vi "Set_DL_Detector.vi"(8 "error in (no error)":errorcluster, 11 "Control-Server in":refnum<class "Control-Server.lvclass">) -> (0 "error out":errorcluster, 3 "Control-Server out":refnum<class "Control-Server.lvclass">)   [LabVIEW 2015, in "Control-Server.lvclass"]
uses:
  Control-Server.lvclass
  Config/config_names_def.ctl
  Delay Line/DelayLine.lvclass
  Delay Line/DelayLineLS4/DelayLineLS4.lvclass
  Delay Line/DelayLineOwis/DelayLineOwis.lvclass
  Detector/Detector.lvclass
  Detector/VIS-IR/VIS-NIR.lvclass
  Detector/UV-VIS/UV-VIS.lvclass
  dependecies/ControlsVIs/Clusters-def/UserEvent.ctl
  dependecies/ControlsVIs/Clusters-def/Message types.ctl
  Message/Message.lvclass
  Message/Message.lvclass/Message.ctl
  GeneralFunctionality/GeneralFunctionality.lvclass/GeneralFunctionality.ctl
  dependecies/ControlsVIs/Clusters-def/list-of-keys-DAQmx-tasks.ctl
  Control-Server.lvclass/Control-Server.ctl
  Detector/Detector.lvclass/Detector.ctl
  Config/Config.lvclass
  GeneralFunctionality/GeneralFunctionality.lvclass
  DAQmxTasks/DAQmxTaskContainer/DAQmxTaskContainer.lvclass
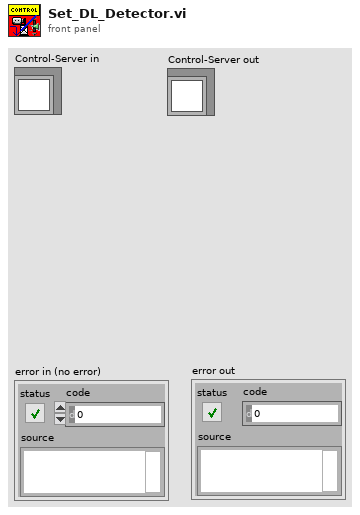
[diagram p1: front panel]
types:
  T1 = typedef "Config.lvclass/config_names_def.ctl" = string
  T2 = typedef "Message types.ctl" = string
  T3 = typedef "UserEvent.ctl" = cluster{"command":string, "data":variant}
  T4 = typedef "DAQmxTaskContainer.lvclass/list-of-keys-DAQmx-tasks.ctl" = string
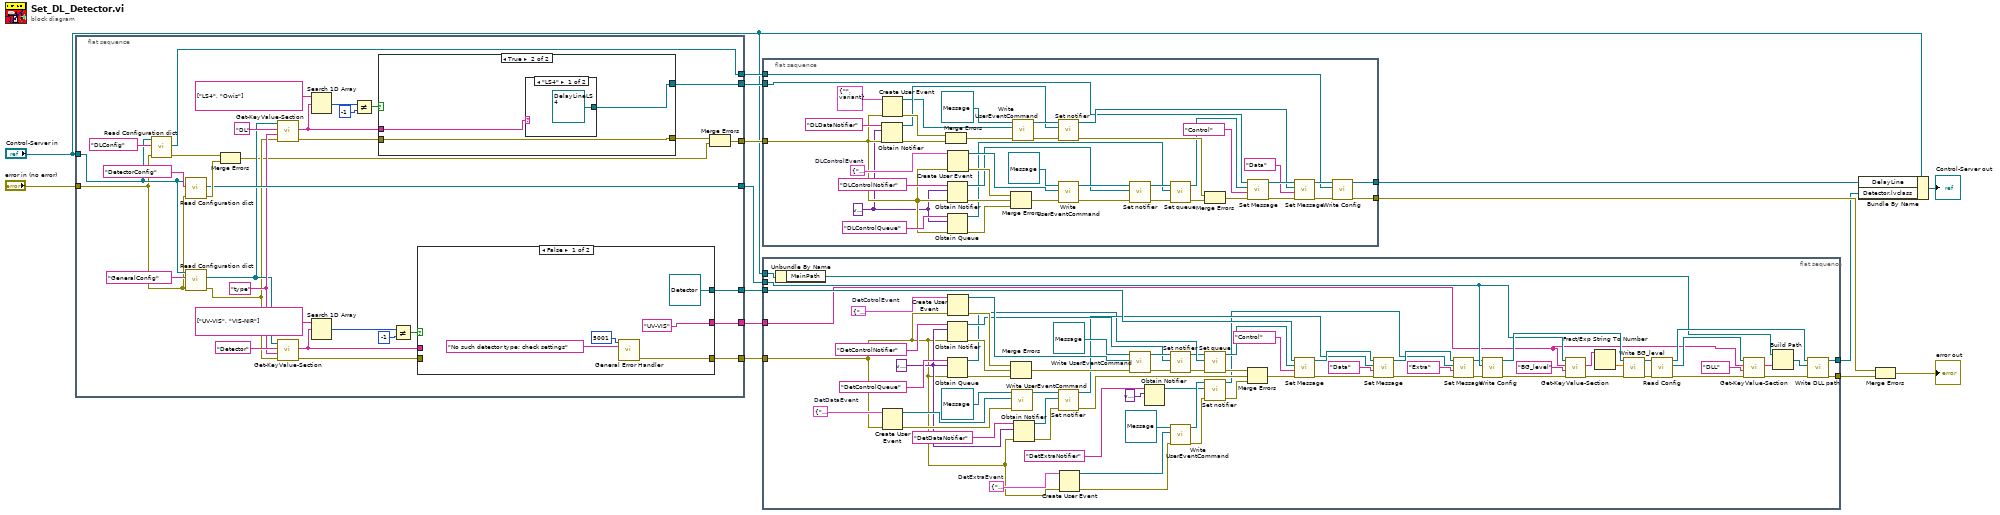
[diagram p0: block diagram]
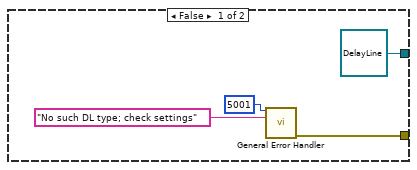
[diagram p2: hidden frame]
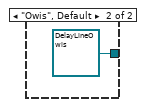
[diagram p3: hidden frame]
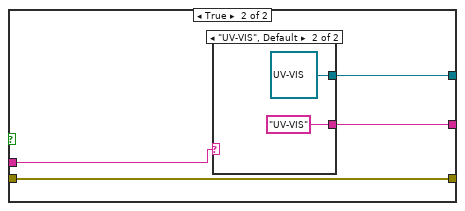
[diagram p4: hidden frame]
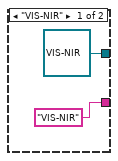
[diagram p5: hidden frame]
diagram:
  n1 = flat-sequence {
    tunnel: "Control-Server in" -> [w32]
    tunnel: "error in (no error)" -> [w31]
    tunnel: [w36] -> w9
    tunnel: [w18] -> w10
    tunnel: [w35] -> w11
    tunnel: [w34] -> w12
    tunnel: [w33] -> w13
    tunnel: [w27] -> w15
    tunnel: [w16] -> w1
    frame #0 {
      w25 = "type" ("Key")
      n2 = call "Read Configuration dict.vi"("error in (no error)"=w31, "Config Name"=T1 "DLConfig", "Control in"=w32) -> ("error out"=w38:errorcluster, "Config"=w36:refnum<class "Config.lvclass">)  [unwired: 6 in, 1 out]
      n3 = call "Read Configuration dict.vi"("error in (no error)"=w31, "Config Name"=T1 "DetectorConfig", "Control in"=w32) -> ("error out"=w37:errorcluster, "Config"=w35:refnum<class "Config.lvclass">)  [unwired: 6 in, 1 out]
      n4 = call "Read Configuration dict.vi"("error in (no error)"=w31, "Config Name"=T1 "GeneralConfig", "Control in"=w32) -> ("error out"=w22:errorcluster, "Config"=w23:refnum<class "Config.lvclass">)  [unwired: 6 in, 1 out]
      n5 = Merge Errors(w38, w37) -> (w20:errorcluster)
      n6 = call-dynamic "Get-KeyValue-Section.vi"("error in (no error)"=w22, "Key"=w25, "Section"="DL", "Config in"=w23) -> ("error out"=w21:errorcluster, "Value"=w17:string)  [unwired: 5 in, 1 out]
      n7 = call-dynamic "Get-KeyValue-Section.vi"("error in (no error)"=w22, "Key"=w25, "Section"="Detector", "Config in"=w23) -> ("error out"=w41:errorcluster, "Value"=w42:string)  [unwired: 5 in, 1 out]
      n8 = Search 1D Array(1D array=string[] ["LS4", "Owis"], element=w17) -> (index of element=w29:i32)  [unwired: 1 in]
      n9 = Search 1D Array(1D array=string[] ["UV-VIS", "VIS-NIR"], element=w42) -> (index of element=w45:i32)  [unwired: 1 in]
      n10 = Not Equal?(x=w29, y=-1) -> (x != y?=w28:bool)
      n11 = case shown="True" w28 {
        tunnel: [w50 w54] -> w19
        tunnel: [refnum<class "DelayLine.lvclass"> refnum ("DelayLine.lvclass") w55] -> w27
        tunnel: w21 -> [_ w54]
        tunnel: w17 -> [_ w53]
        frame False {
          n12 = call <vilib>:"General Error Handler.vi"("[error code] (0)"=5001 ("code"), "[error source] (\" \")"="No such DL type; check settings" ("String to Prepend to source (\"\")")) -> ("error out"=w50:errorcluster)  [unwired: 9 in, 4 out]
        }
        frame True {
          n13 = case shown="\"LS4\"" w53 {
            tunnel: [refnum<class "DelayLineLS4.lvclass"> refnum ("DelayLineLS4.lvclass") refnum<class "DelayLineOwis.lvclass"> refnum ("DelayLineOwis.lvclass")] -> w55
            frame "LS4" {
            }
            frame "Owis", Default {
            }
          }
        }
      }
      n14 = Not Equal?(x=w45, y=-1) -> (x != y?=w43:bool)
      n15 = case shown="False" w43 {
        tunnel: w42 -> [_ w66]
        tunnel: [refnum<class "Detector.lvclass"> refnum ("Detector.lvclass") w64] -> w33
        tunnel: w41 -> [_ w65]
        tunnel: [w59 w65] -> w34
        tunnel: ["UV-VIS" ("Section") w63] -> w16
        frame False {
          n16 = call <vilib>:"General Error Handler.vi"("[error code] (0)"=5001 ("code"), "[error source] (\" \")"="No such detector type; check settings" ("String to Prepend to source (\"\")")) -> ("error out"=w59:errorcluster)  [unwired: 9 in, 4 out]
        }
        frame True {
          n17 = case shown="\"UV-VIS\", Default" w66 {
            tunnel: [refnum<class "VIS-NIR.lvclass"> refnum ("VIS-IR.lvclass") refnum<class "UV-VIS.lvclass"> refnum ("UV-VIS.lvclass")] -> w64
            tunnel: ["VIS-NIR" ("Section") "UV-VIS" ("Section")] -> w63
            frame "VIS-NIR" {
            }
            frame "UV-VIS", Default {
            }
          }
        }
      }
      n18 = Merge Errors(w19, w20) -> (w18:errorcluster)
    }
  }
  n19 = flat-sequence {
    tunnel: w9 -> [w73]
    tunnel: [w112] -> w5
    tunnel: [w111] -> w8
    tunnel: w10 -> [w76]
    tunnel: w15 -> [w72]
    frame #0 {
      w71 = variant
      w106 = cluster{"command":string, "data":variant} {"command"="", "data"=variant}  # DLControlEvent
      n20 = Obtain Notifier(name (unnamed)="DLDataNotifier" ("nom (aucun)"), notification data type=w71, error in (no error)=w76) -> (notifier out=w87:refnum<notifier>, error out=w91:errorcluster)  [unwired: 1 in, 1 out]
      n21 = Create User Event(user event datatype=T3 {"command"="", "data"=variant} ("DLDataEvent"), error in=w76) -> (user event=w86:refnum<user-event>, error out=w92:errorcluster)
      n22 = Merge Errors(w92, w91) -> (w90:errorcluster)
      n23 = Obtain Notifier(name (unnamed)="DLControlNotifier" ("nom (aucun)"), notification data type=w71, error in (no error)=w76) -> (notifier out=w102:refnum<notifier>, error out=w103:errorcluster)  [unwired: 1 in, 1 out]
      n24 = Obtain Queue(name (unnamed)="DLControlQueue", element data type=w71, error in (no error)=w76) -> (queue out=w78:refnum<queue>, error out=w77:errorcluster)  [unwired: 2 in, 1 out]
      n25 = Create User Event(user event datatype=w106, error in=w76) -> (user event=w108:refnum<user-event>, error out=w104:errorcluster)
      n26 = Merge Errors(w104, w103, w77) -> (w101:errorcluster)
      n27 = call "Write UserEventCommand.vi"("error in (no error)"=w90, "UserEventCommand"=w86, "Message en entrée"=refnum<class "Message.lvclass"> refnum ("Message.lvclass")) -> ("error out"=w89:errorcluster, "Message en sortie"=w88:refnum<class "Message.lvclass">)  [unwired: 7 in]
      n28 = call "Set notifier.vi"("error in (no error)"=w89, "notifier"=w87, "Message en entrée"=w88) -> ("error out"=w84:errorcluster, "Message en sortie"=w82:refnum<class "Message.lvclass">)  [unwired: 7 in]
      n29 = call "Write UserEventCommand.vi"("error in (no error)"=w101, "UserEventCommand"=w108, "Message en entrée"=refnum<class "Message.lvclass"> refnum ("Message.lvclass")) -> ("error out"=w105:errorcluster, "Message en sortie"=w109:refnum<class "Message.lvclass">)  [unwired: 7 in]
      n30 = call "Set notifier.vi"("error in (no error)"=w105, "notifier"=w102, "Message en entrée"=w109) -> ("error out"=w79:errorcluster, "Message en sortie"=w80:refnum<class "Message.lvclass">)  [unwired: 7 in]
      n31 = call "Set queue.vi"("error in (no error)"=w79, "queue"=w78, "Message in"=w80) -> ("error out"=w75:errorcluster, "Message out"=w74:refnum<class "Message.lvclass">)  [unwired: 7 in]
      n32 = Merge Errors(w84, w75) -> (w83:errorcluster)
      n33 = call "Set Message.vi"("error in (no error)"=w83, "Message type"=T2 "Control", "Message.lvclass"=w74, "GeneralFunctionality en entrée"=w72) -> ("error out"=w97:errorcluster, "GeneralFunctionality en sortie"=w96:refnum<class "DelayLine.lvclass">)  [unwired: 6 in]
      n34 = call "Set Message.vi"("error in (no error)"=w97, "Message type"=T2 "Data", "Message.lvclass"=w82, "GeneralFunctionality en entrée"=w96) -> ("error out"=w95:errorcluster, "GeneralFunctionality en sortie"=w94:refnum<class "DelayLine.lvclass">)  [unwired: 6 in]
      n35 = call "Write Config.vi"("error in (no error)"=w95, "Config.lvclass"=w73, "GeneralFunctionality en entrée"=w94) -> ("error out"=w111:errorcluster, "GeneralFunctionality en sortie"=w112:refnum<class "DelayLine.lvclass">)  [unwired: 7 in]
    }
  }
  n36 = flat-sequence {
    tunnel: w11 -> [w148]
    tunnel: w12 -> [w134]
    tunnel: w13 -> [w174]
    tunnel: [w115] -> w7
    tunnel: [w118] -> w4
    tunnel: "Control-Server in" -> [w117]
    tunnel: w1 -> [w113]
    frame #0 {
      w135 = cluster{"command":string, "data":variant} {"command"="", "data"=variant}  # DetExtraEvent
      w144 = variant
      w173 = cluster{"command":string, "data":variant} {"command"="", "data"=variant}  # DetDataEvent
      w180 = cluster{"command":string, "data":variant} {"command"="", "data"=variant}  # DetCotrolEvent
      n37 = Unbundle By Name(w117) -> ("MainPath"=w116:path)
      n38 = Create User Event(user event datatype=w173, error in=w134) -> (user event=w169:refnum<user-event>, error out=w168:errorcluster)
      n39 = Obtain Notifier(name (unnamed)="DetControlNotifier" ("nom (aucun)"), notification data type=w144, error in (no error)=w134) -> (notifier out=w176:refnum<notifier>, error out=w177:errorcluster)  [unwired: 1 in, 1 out]
      n40 = Obtain Queue(name (unnamed)="DetControlQueue", element data type=w144, error in (no error)=w134) -> (queue out=w157:refnum<queue>, error out=w156:errorcluster)  [unwired: 2 in, 1 out]
      n41 = Create User Event(user event datatype=w180, error in=w134) -> (user event=w182:refnum<user-event>, error out=w178:errorcluster)
      n42 = Merge Errors(w178, w177, w156) -> (w175:errorcluster)
      n43 = call "Write UserEventCommand.vi"("error in (no error)"=w168, "UserEventCommand"=w169, "Message en entrée"=refnum<class "Message.lvclass"> refnum ("Message.lvclass")) -> ("Message en sortie"=w170:refnum<class "Message.lvclass">)  [unwired: 7 in, 1 out]
      n44 = Obtain Notifier(name (unnamed)="DetDataNotifier" ("nom (aucun)"), notification data type=w144, error in (no error)=w134) -> (notifier out=w166:refnum<notifier>, error out=w167:errorcluster)  [unwired: 1 in, 1 out]
      n45 = call "Set notifier.vi"("error in (no error)"=w167, "notifier"=w166, "Message en entrée"=w170) -> ("error out"=w165:errorcluster, "Message en sortie"=w161:refnum<class "Message.lvclass">)  [unwired: 7 in]
      n46 = Create User Event(user event datatype=w135, error in=w134) -> (user event=w137:refnum<user-event>, error out=w136:errorcluster)
      n47 = call "Write UserEventCommand.vi"("error in (no error)"=w175, "UserEventCommand"=w182, "Message en entrée"=refnum<class "Message.lvclass"> refnum ("Message.lvclass")) -> ("error out"=w179:errorcluster, "Message en sortie"=w183:refnum<class "Message.lvclass">)  [unwired: 7 in]
      n48 = Obtain Notifier(name (unnamed)="DetExtraNotifier" ("nom (aucun)"), notification data type=variant) -> (notifier out=w129:refnum<notifier>)  [unwired: 2 in, 2 out]
      n49 = call "Set notifier.vi"("error in (no error)"=w179, "notifier"=w176, "Message en entrée"=w183) -> ("error out"=w155:errorcluster, "Message en sortie"=w153:refnum<class "Message.lvclass">)  [unwired: 7 in]
      n50 = call "Write UserEventCommand.vi"("error in (no error)"=w136, "UserEventCommand"=w137, "Message en entrée"=refnum<class "Message.lvclass"> refnum ("Message.lvclass")) -> ("error out"=w132:errorcluster, "Message en sortie"=w133:refnum<class "Message.lvclass">)  [unwired: 7 in]
      n51 = call "Set queue.vi"("error in (no error)"=w155, "queue"=w157, "Message in"=w153) -> ("error out"=w154:errorcluster, "Message out"=w152:refnum<class "Message.lvclass">)  [unwired: 7 in]
      n52 = call "Set notifier.vi"("error in (no error)"=w132, "notifier"=w129, "Message en entrée"=w133) -> ("error out"=w128:errorcluster, "Message en sortie"=w139:refnum<class "Message.lvclass">)  [unwired: 7 in]
      n53 = Merge Errors(w154, w165, w128) -> (w164:errorcluster)
      n54 = call "Set Message.vi"("error in (no error)"=w164, "Message type"=T2 "Control", "Message.lvclass"=w152, "GeneralFunctionality en entrée"=w174) -> ("error out"=w162:errorcluster, "GeneralFunctionality en sortie"=w163:refnum<class "Detector.lvclass">)  [unwired: 6 in]
      n55 = call "Set Message.vi"("error in (no error)"=w162, "Message type"=T2 "Data", "Message.lvclass"=w161, "GeneralFunctionality en entrée"=w163) -> ("error out"=w143:errorcluster, "GeneralFunctionality en sortie"=w140:refnum<class "Detector.lvclass">)  [unwired: 6 in]
      n56 = call "Set Message.vi"("error in (no error)"=w143, "Message type"=T2 "Extra", "Message.lvclass"=w139, "GeneralFunctionality en entrée"=w140) -> ("error out"=w142:errorcluster, "GeneralFunctionality en sortie"=w141:refnum<class "Detector.lvclass">)  [unwired: 6 in]
      n57 = call "Write Config.vi"("error in (no error)"=w142, "Config.lvclass"=w148, "GeneralFunctionality en entrée"=w141) -> ("error out"=w150:errorcluster, "GeneralFunctionality en sortie"=w151:refnum<class "Detector.lvclass">)  [unwired: 7 in]
      n58 = call-dynamic "Get-KeyValue-Section.vi"("error in (no error)"=w150, "Key"="BG_level", "Section"=w113, "Config in"=w148) -> ("error out"=w149:errorcluster, "Value"=w146:string)  [unwired: 5 in, 1 out]
      n59 = Fract/Exp String To Number(string=w146) -> (number=w145:dbl)  [unwired: 3 in, 1 out]
      n60 = call-dynamic "Write BG_level.vi"("error in (no error)"=w149, "BG_level"=w145, "Detector in"=w151) -> ("error out"=w114:errorcluster, "Detector out"=w119:refnum<class "Detector.lvclass">)  [unwired: 7 in]
      n61 = call "Read Config.vi"("error in (no error)"=w114, "GeneralFunctionality en entrée"=w119) -> ("error out"=w125:errorcluster, "Config.lvclass"=w123:refnum<class "Config.lvclass">, "GeneralFunctionality en sortie"=w126:refnum<class "Detector.lvclass">)  [unwired: 7 in]
      n62 = call-dynamic "Get-KeyValue-Section.vi"("error in (no error)"=w125, "Key"=T4 "DLL", "Section"=w113, "Config in"=w123) -> ("error out"=w124:errorcluster, "Value"=w122:string)  [unwired: 5 in, 1 out]
      n63 = Build Path(base path=w116, name or relative path=w122) -> (appended path=w120:path)
      n64 = call "Write DLL path.vi"("error in (no error)"=w124, "DLL path"=w120, "Detector in"=w126) -> ("error out"=w115:errorcluster, "Detector out"=w118:refnum<class "Detector.lvclass">)  [unwired: 7 in]
    }
  }
  n65 = Bundle By Name(cluster="Control-Server in", "DelayLine"=w5, "Detector.lvclass"=w4) -> (→"Control-Server out":refnum<class "Control-Server.lvclass">)
  n66 = Merge Errors(w8, w7) -> (→"error out":errorcluster)
